vi "MV main 1.0.vi"() -> ()   [LabVIEW 2009, in "Millennia V.lvclass"]
uses:
  Millennia V.lvclass
panel:
  out "Error":bool caption="Shut Down"
  out "on?":bool
  in  "setpower":bool
  in  "power ctrl":dbl=0.2 min=0.2 max=5.0 step=0.01 format="%.2g"
  out "Power (W)":dbl(knob) scale=0.0..5.0
  out "Warmed up":dbl(slide) scale=0.0..100.0
  in  "findMV":bool
  in  "exit":bool
  out "Millennia V found":bool
  in  "warm-up/on":bool
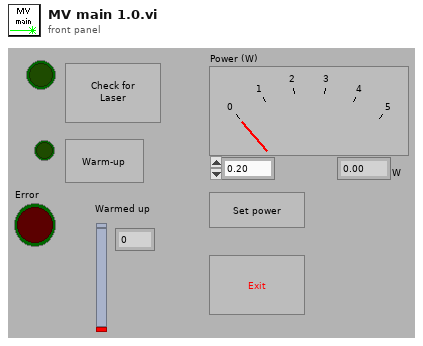
[diagram p1: front panel]
types:
  T1 = typedef "Millennia V.lvclass/MV status.ctl" = cluster{"Millennia V found":bool, "on?":bool, "Error":bool, "Warmed up":T2}
  T2 = typedef "Millennia V.lvclass/MV warmed up.ctl" = dbl
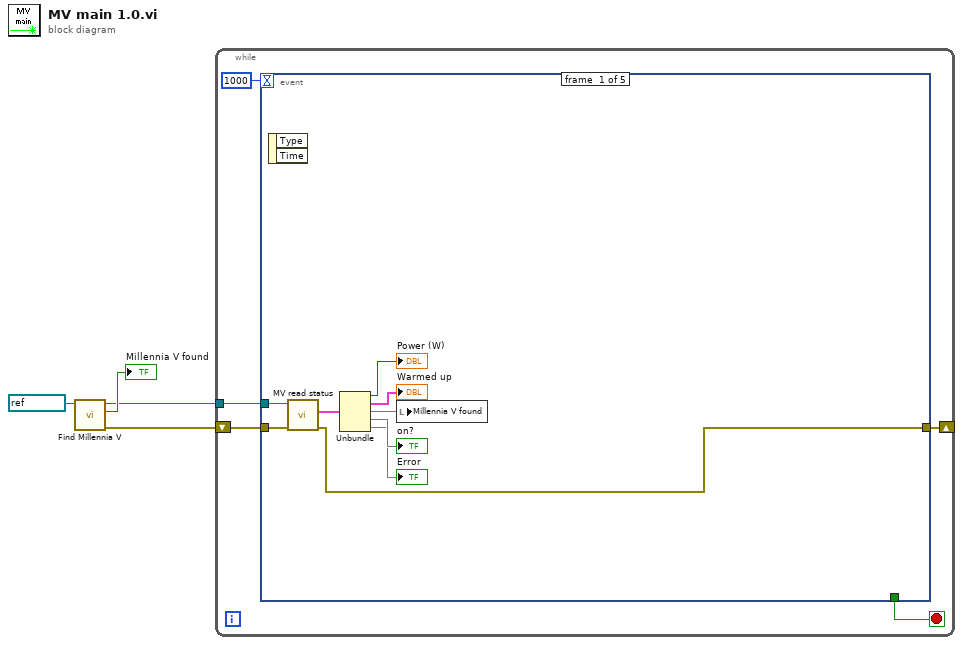
[diagram p0: block diagram]
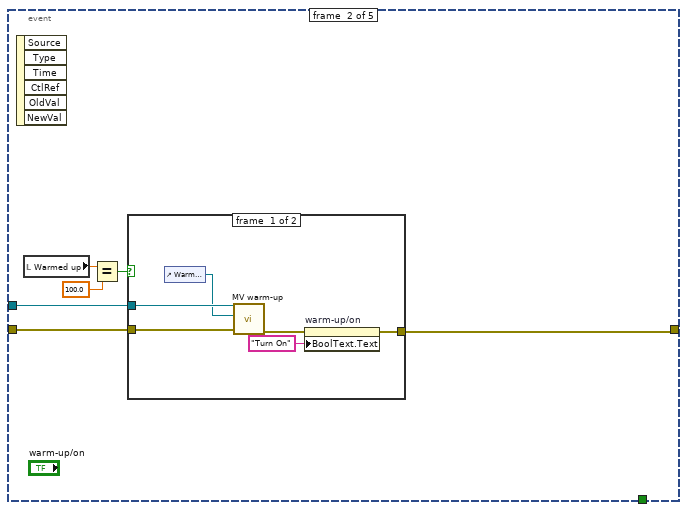
[diagram p2: hidden frame]
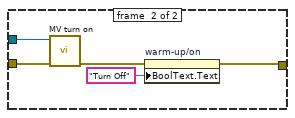
[diagram p3: hidden frame]
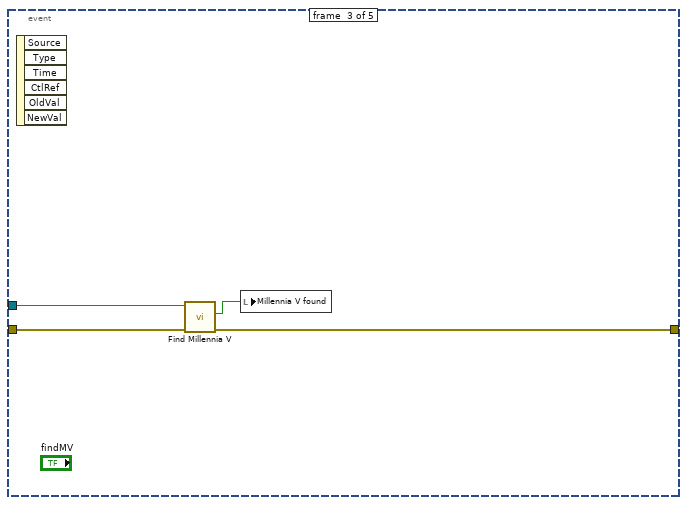
[diagram p4: hidden frame]
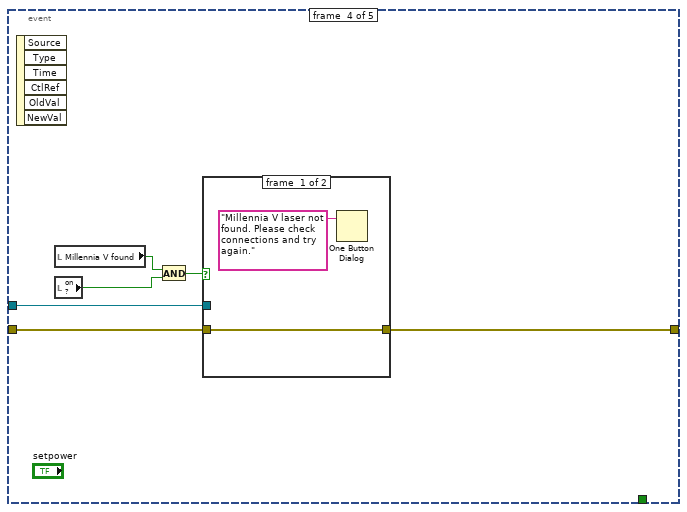
[diagram p5: hidden frame]
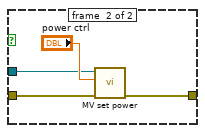
[diagram p6: hidden frame]
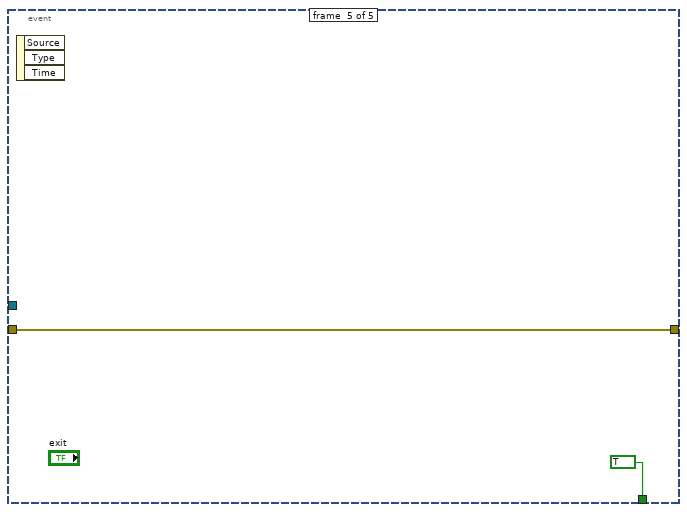
[diagram p7: hidden frame]
diagram:
  n1 = call "Find Millennia V.vi"("VISA resource name"=refnum<visa-resource-name> "COM1") -> ("error out"=w2:errorcluster, "Millennia V found"=→"Millennia V found":bool, "VISA resource name out"=w1:refnum<visa-resource-name>)  [unwired: 8 in]
  n2 = while {
    shift-right: [w7] -> _
    shift-left: w2 -> [w8]
    tunnel: w1 -> [w6]
    stop <- w9 stop-if-true
    n3 = event shown="[1] \"warm-up/on\": Value Change" {
      selector: _ -> [_ _ _ _ _]
      dyn-events: _ -> [_ _ _ _ _]
      timeout: 1000 -> [_ _ _ _ _]
      tunnel: [_ _ _ _ TRUE] -> w9
      tunnel: w8 -> [w17 w23 w39 w42 w52]
      tunnel: [w10 w22 w38 w40 w52] -> w7
      tunnel: w6 -> [w18 w24 w36 w41 _]
      event #0 {
        n4 = event-data() -> ()  [unwired: 1 in, 2 out]
        n5 = call "MV read status.vi"("error in (no error)"=w17, "VISA resource name"=w18) -> ("error out"=w10:errorcluster, "status cluster"=w16:cluster{"Power (W)":i32, "status indicators":T1})  [unwired: 7 in, 1 out]
        n6 = Unbundle(w16) -> (→"Power (W)":i32, →"Warmed up":T1, w13, →"on?", →"Error")
        n7 = local write "Millennia V found"(w13) -> ()
      }
      event #1 {
        n8 = event-data() -> ()  [unwired: 1 in, 6 out]
        n9 = local read "Warmed up"() -> (w20:dbl)
        n10 = Equal?(x=w20, y=100.0) -> (x = y?=w21:bool)
        n11 = case shown="True" w21 {
          tunnel: w24 -> [w30 w35]
          tunnel: w23 -> [w29 w34]
          tunnel: [w26 w32] -> w22
          frame #0 {
            n12 = control-ref of="Warmed up"() -> (w28:refnum<vi>)
            n13 = call "MV warm-up.vi"("error in (no error)"=w29, "slide indicator reference"=w28, "VISA resource name"=w30) -> ("error out"=w27:errorcluster)  [unwired: 7 in, 1 out]
            n14 = property on="warm-up/on" class="Bool"(error in=w27, "BoolText.Text"="Turn On" ("Boolean Text.Text")) -> (error out=w26:errorcluster)  [unwired: 1 in, 1 out]
          }
          frame #1 {
            n15 = call "MV turn on.vi"("error in (no error)"=w34, "VISA resource name"=w35) -> ("error out"=w33:errorcluster)  [unwired: 8 in, 1 out]
            n16 = property on="warm-up/on" class="Bool"(error in=w33, "BoolText.Text"="Turn Off" ("Boolean Text.Text")) -> (error out=w32:errorcluster)  [unwired: 1 in, 1 out]
          }
        }
      }
      event #2 {
        n17 = event-data() -> ()  [unwired: 1 in, 6 out]
        n18 = call "Find Millennia V.vi"("error in (no error)"=w39, "VISA resource name"=w36) -> ("error out"=w38:errorcluster, "Millennia V found"=w37:bool)  [unwired: 7 in, 1 out]
        n19 = local write "Millennia V found"(w37) -> ()
      }
      event #3 {
        n20 = event-data() -> ()  [unwired: 1 in, 6 out]
        n21 = local read "Millennia V found"() -> (w45:bool)
        n22 = local read "on?"() -> (w44:bool)
        n23 = And(x=w45, y=w44) -> (x .and. y?=w43:bool)
        n24 = case shown="False" w43 {
          tunnel: w42 -> [w47 w49]
          tunnel: w41 -> [_ w50]
          tunnel: [w47 w48] -> w40
          frame #0 {
            n25 = One Button Dialog(message="Millennia V laser not found. Please check connections and try again.") -> ()  [unwired: 1 in, 1 out]
          }
          frame #1 {
            n26 = call "MV set power.vi"("error in (no error)"=w49, "power (W)"="power ctrl", "VISA resource name"=w50) -> ("error out"=w48:errorcluster)  [unwired: 7 in, 1 out]
          }
        }
      }
      event #4 {
        n27 = event-data() -> ()  [unwired: 1 in, 3 out]
      }
    }
  }
